vi "五参数水样测试.vi"(11 "启动参数":T1={"测量模式"=enum."水样测试", "数据标记表"="N", "测量时间"=3.0}) -> ()   [LabVIEW 2016, in "斯坦道多参数.lvlib"]
panel:
  out "枚举":T2(ring)
  out "状态":string
  out "数值":i32
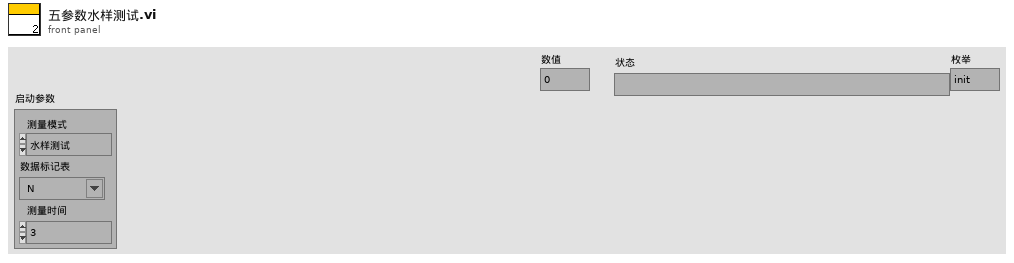
[diagram p1: front panel]
types:
  T1 = cluster{"测量模式":enum16{"待机", "水样测试", "标样核查", "零点核查", "跨度核查", "空白测试", "平行样测试", "加标回收", "空白校准", "标样校准", "初始化（清洗）"}, "数据标记表":string, "测量时间":dbl}
  T2 = enum16{"init", "开机", "启动测量", "读取测量值", "存储数据", "关闭测量", "关机", "结束"}
  T3 = cluster{"时间标识":timestamp, "设备":string, "日志信息":string, "流程参数":string}
  T4 = cluster{"系统时间":timestamp, "工作状态":u16, "测量模式":u16, "告警代码":enum16{"无告警", "缺试剂告警", "缺水样告警", "缺蒸馏水告警", "缺标液告警", "仪表漏液告警", "标定异常告警", "超量程告警", "加热异常", "低试剂预警", "超上限告警", "超下限告警", "仪表内部其他异常", "滴定异常告警", "电极异常告警", "量程切换告警", "参数设置告警", "PH电极电位异常", "电导率电极异常", "浊度光度异常", "溶解氧电极异常", "溶解氧光强异常", "温度异常告警", "PH异常告警", "溶解氧异常告警", "电导率异常告警", "浊度异常告警", "叶绿素异常告警", "藻密度异常告警", "蓝绿藻异常告警", "ORP异常告警", "氨氮异常告警", "清洁刷异常告警", "SD卡异常告警", "蓝牙异常告警", "Wifi异常告警", "流程异常告警"}, "故障代码":enum16{"无故障", "电机故障", "温度故障", "通讯故障", "滴定故障"}, "日志代码":u16, "软件版本":string}
  T5 = enum16{"待机", "水样测试", "标样核查", "零点核查", "跨度核查", "空白测试", "平行样测试", "加标回收", "空白校准", "标样校准", "初始化（清洗）"}
  T6 = cluster{"水温":dbl, "pH":dbl, "DO":dbl, "Cond":dbl, "Turb":dbl, "叶绿素":dbl, "藻密度":dbl, "蓝绿藻":dbl, "ORP":dbl, "NH3N":dbl}
  T7 = cluster{"数据标记表":string, "测量模式":enum16{"待机", "水样测试", "标样核查", "零点核查", "跨度核查", "空白测试", "平行样测试", "加标回收", "空白校准", "标样校准", "初始化（清洗）"}, "database":string}
  T8 = cluster{"因子编码":string, "单位":string, "标样参考值":sgl, "水样数据时间":timestamp, "水样实测值":sgl, "水样数据标识":string, "K":sgl, "B":sgl, "T":sgl, "H":sgl, "水深":sgl, "探头温度":sgl}
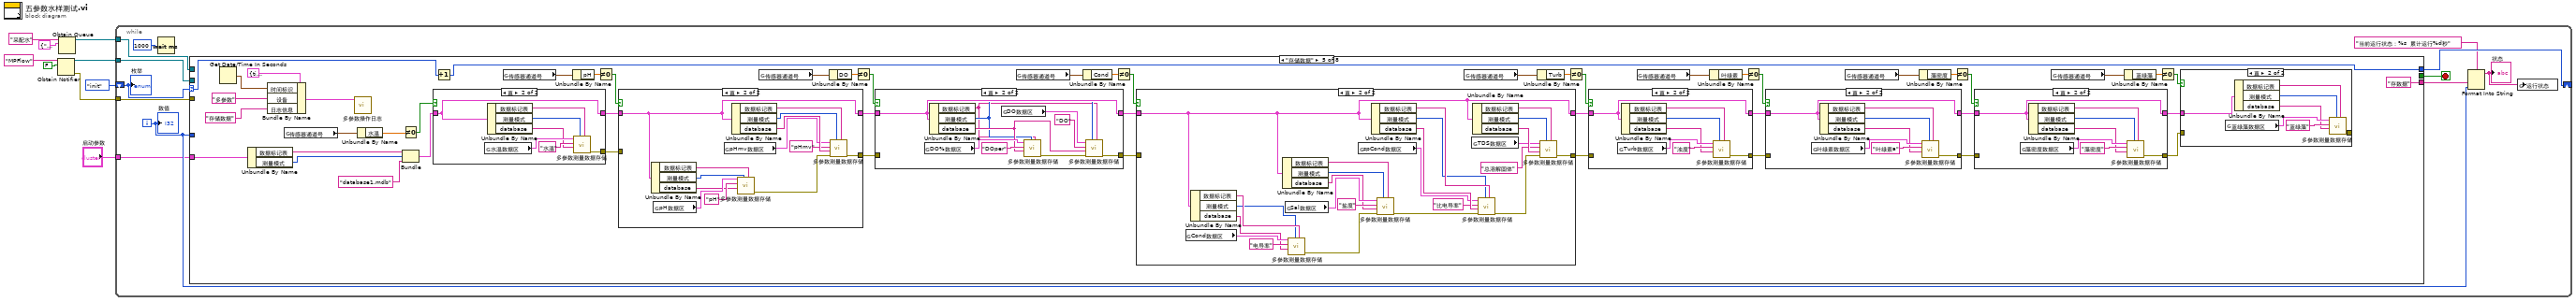
[diagram p0: block diagram]
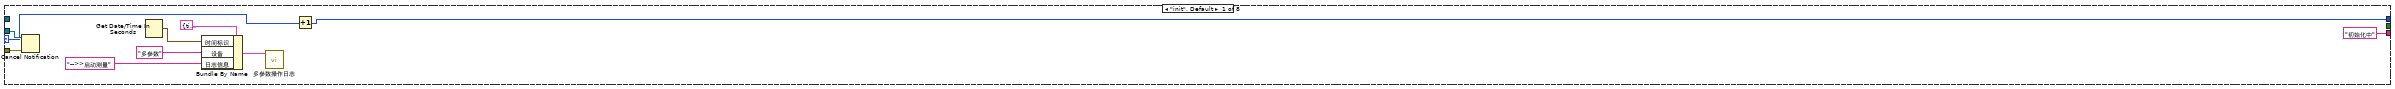
[diagram p2: hidden frame]
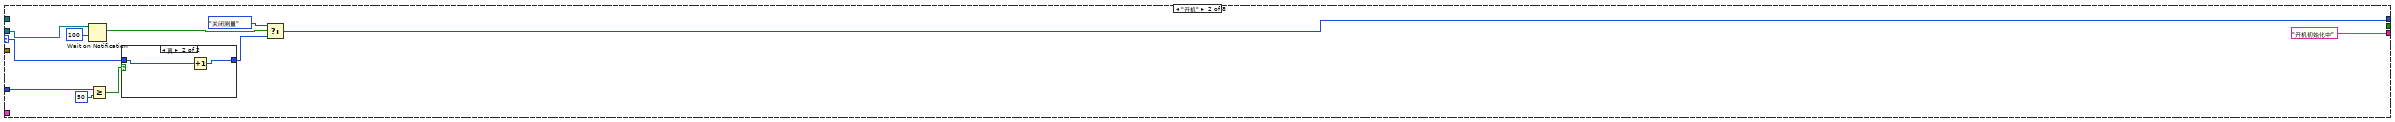
[diagram p3: hidden frame]
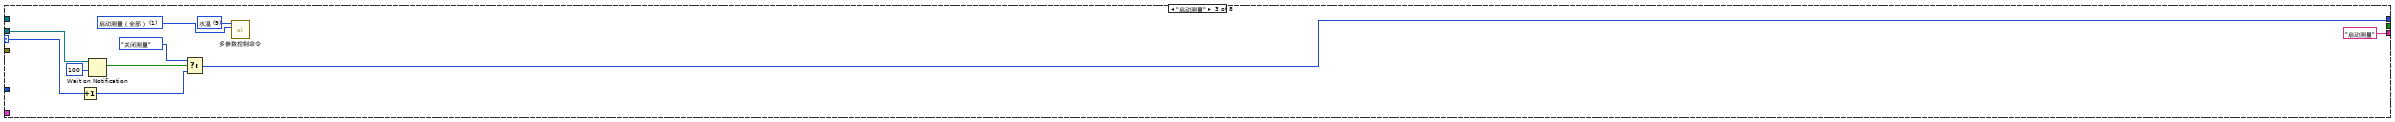
[diagram p5: hidden frame]
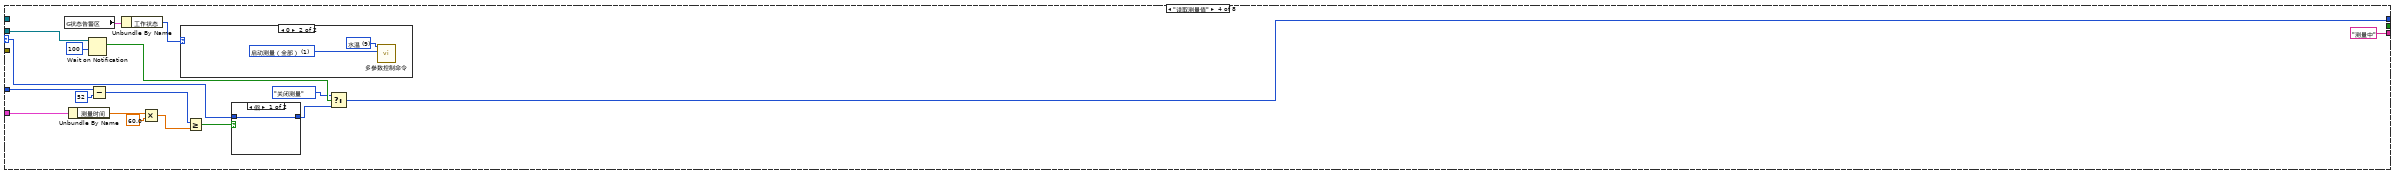
[diagram p6: hidden frame]
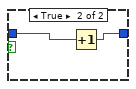
[diagram p8: hidden frame]
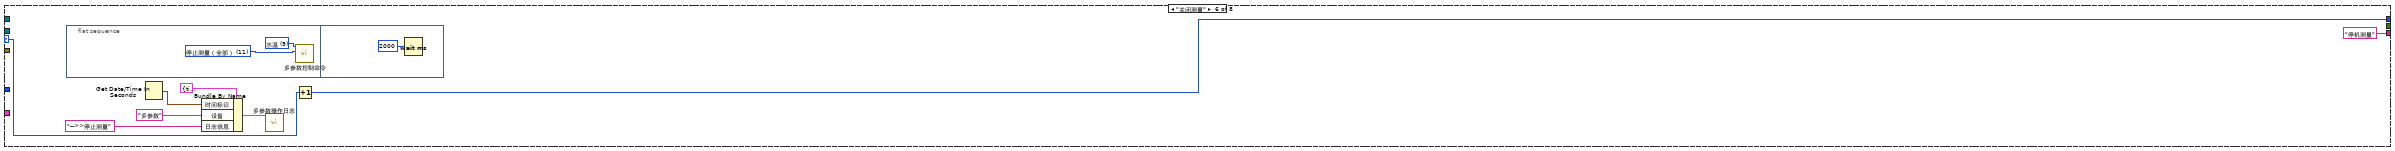
[diagram p17: hidden frame]
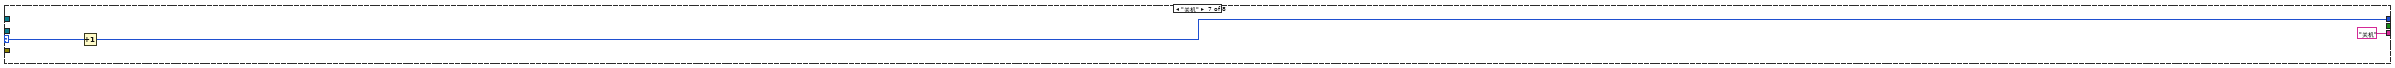
[diagram p18: hidden frame]
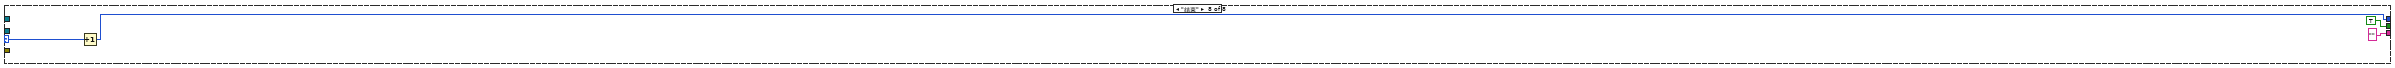
[diagram p19: hidden frame]
diagram:
  n1 = Obtain Notifier(name (unnamed)="MPFlow" ("名称（未命名）"), notification data type=FALSE) -> (notifier out=w6:refnum<notifier>, error out=w5:errorcluster)  [unwired: 2 in, 1 out]
  n2 = Obtain Queue(name (unnamed)="采配水" ("名称（未命名）"), element data type=cluster{"命令":string, "数据":variant} {"命令"="", "数据"=variant}) -> (queue out=w1:refnum<queue>)  [unwired: 3 in, 2 out]
  n3 = while {
    shift-right: [w17] -> _
    shift-left: T2."init" ("枚举") -> [w21]
    tunnel: w6 -> [w19]
    tunnel: w5 -> [w18]
    tunnel: "启动参数" -> [w11]
    tunnel: w1 -> [w10]
    i -> [w13]
    stop <- w20 stop-if-true
    n4 = Wait (ms)(milliseconds to wait=u32 1000 ("等待时间（毫秒）")) -> ()  [unwired: 1 out]
    n5 = case shown="\"存储数据\"" w21 {
      selector: w21 -> [w29 w42 w55 w73 w129 w227 w233 w236]
      tunnel: [_ _ _ _ _ _ _ TRUE] -> w20
      tunnel: w19 -> [w31 w37 w54 w70 _ _ _ _]
      tunnel: w18 -> [w30 _ _ _ _ _ _ _]
      tunnel: [w28 w35 w51 w68 w128 w226 w232 w235] -> w17
      tunnel: w13 -> [_ w41 _ w60 _ _ _ _]
      tunnel: ["初始化中" ("状态") "开机初始化中" ("状态") "启动测量" ("状态") "测量中" ("状态") "存数据" ("状态") "停机测量" ("状态") "关机" ("状态") "" ("状态")] -> w14
      tunnel: w11 -> [_ _ _ w64 w126 _ _ _]
      tunnel: w10 -> [_ _ _ _ _ _ _ _]
      frame "init", Default {
        n6 = Cancel Notification(0:w31, 3:w30) -> ()  [unwired: 3 out]
        n7 = Get Date/Time In Seconds() -> (seconds since 1Jan1904=w25:timestamp)
        n8 = Bundle By Name(cluster=T3 {"时间标识"=timestamp(0 s since 1904-01-01), "设备"="", "日志信息"="", "流程参数"=""} ("data in"), "时间标识"=w25, "设备"="多参数", "日志信息"="-->>启动测量") -> (w24:T3)
        n9 = call "多参数操作日志.vi"("data in"=w24) -> ()  [unwired: 10 in, 1 out]
        n10 = Increment(x=w29) -> (x+1=w28:T2)
      }
      frame "开机" {
        n11 = Wait on Notification(notifier=w37, timeout in ms (-1)=100 ("超时毫秒(-1)")) -> (notification=w38:bool)  [unwired: 2 in, 3 out]
        n12 = Greater Or Equal?(x=w41, y=50) -> (x >= y?=w39:bool)
        n13 = case shown="真" w39 {
          tunnel: w42 -> [w43 w45]
          tunnel: [w43 w44] -> w36
          frame False {
          }
          frame True {
            n14 = Increment(x=w45) -> (x+1=w44:T2)
          }
        }
        n15 = Select(t=T2."关闭测量" ("枚举"), s=w38, f=w36) -> (s? t:f=w35:T2)
      }
      frame "启动测量" {
        w46 = u16 1 items=["启动测量（全部）"=1, "初始化（清洗）"=10, "停止测量（全部）"=11, "校时"=13, "启动测量（单个传感器）"=19, "停止测量（单个传感器）"=20] ("控制命令")
        w47 = u16 9 items=["氨氮"=3, "水温"=9, "pH值"=10, "溶解氧"=11, "电导率"=12, "浊度"=13, "叶绿素a"=14, "藻密度"=15, "蓝绿藻"=16, "氧化还原电位"=17, "溶解氧%"=18, "盐度"=19] ("站号")
        n16 = Increment(x=w55) -> (x+1=w52:T2)
        n17 = Wait on Notification(notifier=w54, timeout in ms (-1)=100 ("超时毫秒(-1)")) -> (notification=w53:bool)  [unwired: 2 in, 3 out]
        n18 = Select(t=T2."关闭测量" ("枚举"), s=w53, f=w52) -> (s? t:f=w51:T2)
        n19 = call "多参数控制命令.vi"("控制命令"=w46, "站号"=w47) -> ()  [unwired: 9 in, 1 out]
      }
      frame "读取测量值" {
        n20 = global read "多参数全局变量.vi" "状态告警区"() -> (w57:T4)
        n21 = Unbundle By Name(w64) -> ("测量时间"=w63:dbl)
        n22 = Wait on Notification(notifier=w70, timeout in ms (-1)=100 ("超时毫秒(-1)")) -> (notification=w71:bool)  [unwired: 2 in, 3 out]
        n23 = Subtract(x=w60, y=52) -> (x-y=w59:i32)
        n24 = Unbundle By Name(w57) -> ("工作状态"=w56:u16)
        n25 = Multiply(x=w63, y=60.0) -> (x*y=w61:dbl)
        n26 = case shown="0" w56 {
          frame Default {
          }
          frame 0 {
            w74 = u16 1 items=["启动测量（全部）"=1, "初始化（清洗）"=10, "停止测量（全部）"=11, "校时"=13, "启动测量（单个传感器）"=19, "停止测量（单个传感器）"=20] ("控制命令")
            w75 = u16 9 items=["氨氮"=3, "水温"=9, "pH值"=10, "溶解氧"=11, "电导率"=12, "浊度"=13, "叶绿素a"=14, "藻密度"=15, "蓝绿藻"=16, "氧化还原电位"=17, "溶解氧%"=18, "盐度"=19] ("站号")
            n27 = call "多参数控制命令.vi"("控制命令"=w74, "站号"=w75) -> ()  [unwired: 9 in, 1 out]
          }
        }
        n28 = Greater Or Equal?(x=w59, y=w61) -> (x >= y?=w72:bool)
        n29 = case shown="假" w72 {
          tunnel: w73 -> [w76 w78]
          tunnel: [w76 w77] -> w69
          frame False {
          }
          frame True {
            n30 = Increment(x=w78) -> (x+1=w77:T2)
          }
        }
        n31 = Select(t=T2."关闭测量" ("枚举"), s=w71, f=w69) -> (s? t:f=w68:T2)
      }
      frame "存储数据" {
        n32 = Get Date/Time In Seconds() -> (seconds since 1Jan1904=w97:timestamp)
        n33 = Unbundle By Name(w126) -> ("数据标记表"=w105:string, "测量模式"=w104:T5)
        n34 = Bundle By Name(cluster=T3 {"时间标识"=timestamp(0 s since 1904-01-01), "设备"="", "日志信息"="", "流程参数"=""} ("data in"), "时间标识"=w97, "设备"="多参数", "日志信息"="存储数据") -> (w96:T3)
        n35 = global read "多参数全局变量.vi" "传感器通道号"() -> (w121:T6)
        n36 = call "多参数操作日志.vi"("data in"=w96) -> ()  [unwired: 10 in, 1 out]
        n37 = Unbundle By Name(w121) -> ("水温"=w120:dbl)
        n38 = Not Equal To 0?(x=w120) -> (x != 0?=w119:bool)
        n39 = Bundle("数据标记表"=w105, "测量模式"=w104, "database"="database1.mdb") -> (w103:T7)  [unwired: 1 in]
        n40 = case shown="真" w119 {
          tunnel: [_ w217] -> w125
          tunnel: w103 -> [w212 w216]
          tunnel: [w212 w216] -> w102
          frame False {
          }
          frame True {
            n41 = global read "多参数全局变量.vi" "水温数据区"() -> (w219:T8)
            n42 = Unbundle By Name(w216) -> ("数据标记表"=w215:string, "测量模式"=w214:T5, "database"=w213:string)
            n43 = call "多参数测量数据存储.vi"("数据标记表"=w215, "测量模式"=w214, "database"=w213, "table输入"="水温", "data in"=w219) -> ("error out"=w217:errorcluster)  [unwired: 6 in]
          }
        }
        n44 = Increment(x=w129) -> (x+1=w128:T2)
        n45 = global read "多参数全局变量.vi" "传感器通道号"() -> (w114:T6)
        n46 = Unbundle By Name(w114) -> ("pH"=w113:dbl)
        n47 = Not Equal To 0?(x=w113) -> (x != 0?=w118:bool)
        n48 = case shown="真" w118 {
          tunnel: w125 -> [_ _]
          tunnel: [_ w201] -> w124
          tunnel: w102 -> [w198 w206]
          tunnel: [w198 w206] -> w100
          frame False {
          }
          frame True {
            n49 = Unbundle By Name(w206) -> ("数据标记表"=w209:string, "测量模式"=w208:T5, "database"=w207:string)
            n50 = global read "多参数全局变量.vi" "pH数据区"() -> (w211:T8)
            n51 = global read "多参数全局变量.vi" "pHmv数据区"() -> (w200:T8)
            n52 = Unbundle By Name(w206) -> ("数据标记表"=w205:string, "测量模式"=w204:T5, "database"=w203:string)
            n53 = call "多参数测量数据存储.vi"("数据标记表"=w209, "测量模式"=w208, "database"=w207, "table输入"="pH", "data in"=w211) -> ("error out"=w202:errorcluster)  [unwired: 6 in]
            n54 = call "多参数测量数据存储.vi"("数据标记表"=w205, "测量模式"=w204, "error in (no error)"=w202, "database"=w203, "table输入"="pHmv", "data in"=w200) -> ("error out"=w201:errorcluster)  [unwired: 5 in]
          }
        }
        n55 = global read "多参数全局变量.vi" "传感器通道号"() -> (w112:T6)
        n56 = Unbundle By Name(w112) -> ("DO"=w111:dbl)
        n57 = Not Equal To 0?(x=w111) -> (x != 0?=w117:bool)
        n58 = case shown="真" w117 {
          tunnel: w124 -> [_ _]
          tunnel: [_ w194] -> w123
          tunnel: [w187 w191] -> w101
          tunnel: w100 -> [w187 w191]
          frame False {
          }
          frame True {
            n59 = global read "多参数全局变量.vi" "DO%数据区"() -> (w193:T8)
            n60 = Unbundle By Name(w191) -> ("数据标记表"=w188:string, "测量模式"=w189:T5, "database"=w190:string)
            n61 = global read "多参数全局变量.vi" "DO数据区"() -> (w195:T8)
            n62 = call "多参数测量数据存储.vi"("数据标记表"=w188, "测量模式"=w189, "database"=w190, "table输入"="DOper", "data in"=w193) -> ("error out"=w197:errorcluster)  [unwired: 6 in]
            n63 = call "多参数测量数据存储.vi"("数据标记表"=w188, "测量模式"=w189, "error in (no error)"=w197, "database"=w190, "table输入"="DO", "data in"=w195) -> ("error out"=w194:errorcluster)  [unwired: 5 in]
          }
        }
        n64 = global read "多参数全局变量.vi" "传感器通道号"() -> (w110:T6)
        n65 = Unbundle By Name(w110) -> ("Cond"=w109:dbl)
        n66 = Not Equal To 0?(x=w109) -> (x != 0?=w116:bool)
        n67 = case shown="真" w116 {
          tunnel: w123 -> [_ _]
          tunnel: [_ w166] -> w122
          tunnel: w101 -> [w161 w175]
          tunnel: [w161 w175] -> w99
          frame False {
          }
          frame True {
            n68 = global read "多参数全局变量.vi" "Cond数据区"() -> (w186:T8)
            n69 = Unbundle By Name(w175) -> ("数据标记表"=w180:string, "测量模式"=w179:T5, "database"=w181:string)
            n70 = Unbundle By Name(w175) -> ("数据标记表"=w178:string, "测量模式"=w177:T5, "database"=w176:string)
            n71 = global read "多参数全局变量.vi" "Sal数据区"() -> (w183:T8)
            n72 = call "多参数测量数据存储.vi"("数据标记表"=w180, "测量模式"=w179, "database"=w181, "table输入"="电导率", "data in"=w186) -> ("error out"=w184:errorcluster)  [unwired: 6 in]
            n73 = global read "多参数全局变量.vi" "spCond数据区"() -> (w165:T8)
            n74 = Unbundle By Name(w175) -> ("数据标记表"=w174:string, "测量模式"=w173:T5, "database"=w172:string)
            n75 = call "多参数测量数据存储.vi"("数据标记表"=w178, "测量模式"=w177, "error in (no error)"=w184, "database"=w176, "table输入"="盐度", "data in"=w183) -> ("error out"=w171:errorcluster)  [unwired: 5 in]
            n76 = global read "多参数全局变量.vi" "TDS数据区"() -> (w164:T8)
            n77 = Unbundle By Name(w175) -> ("数据标记表"=w167:string, "测量模式"=w168:T5, "database"=w169:string)
            n78 = call "多参数测量数据存储.vi"("数据标记表"=w174, "测量模式"=w173, "error in (no error)"=w171, "database"=w172, "table输入"="比电导率", "data in"=w165) -> ("error out"=w170:errorcluster)  [unwired: 5 in]
            n79 = call "多参数测量数据存储.vi"("数据标记表"=w167, "测量模式"=w168, "error in (no error)"=w170, "database"=w169, "table输入"="总溶解固体", "data in"=w164) -> ("error out"=w166:errorcluster)  [unwired: 5 in]
          }
        }
        n80 = global read "多参数全局变量.vi" "传感器通道号"() -> (w108:T6)
        n81 = Unbundle By Name(w108) -> ("Turb"=w107:dbl)
        n82 = Not Equal To 0?(x=w107) -> (x != 0?=w115:bool)
        n83 = case shown="真" w115 {
          tunnel: w122 -> [_ _]
          tunnel: w99 -> [w153 w154]
          tunnel: [_ w155] -> w90
          tunnel: [w153 w154] -> w89
          frame False {
          }
          frame True {
            n84 = global read "多参数全局变量.vi" "Turb数据区"() -> (w160:T8)
            n85 = Unbundle By Name(w154) -> ("数据标记表"=w156:string, "测量模式"=w157:T5, "database"=w158:string)
            n86 = call "多参数测量数据存储.vi"("数据标记表"=w156, "测量模式"=w157, "database"=w158, "table输入"="浊度", "data in"=w160) -> ("error out"=w155:errorcluster)  [unwired: 6 in]
          }
        }
        n87 = global read "多参数全局变量.vi" "传感器通道号"() -> (w92:T6)
        n88 = Unbundle By Name(w92) -> ("叶绿素"=w93:dbl)
        n89 = Not Equal To 0?(x=w93) -> (x != 0?=w91:bool)
        n90 = case shown="真" w91 {
          tunnel: w90 -> [_ _]
          tunnel: w89 -> [w145 w146]
          tunnel: [_ w147] -> w85
          tunnel: [w145 w146] -> w84
          frame False {
          }
          frame True {
            n91 = global read "多参数全局变量.vi" "叶绿素数据区"() -> (w152:T8)
            n92 = Unbundle By Name(w146) -> ("数据标记表"=w148:string, "测量模式"=w149:T5, "database"=w150:string)
            n93 = call "多参数测量数据存储.vi"("数据标记表"=w148, "测量模式"=w149, "database"=w150, "table输入"="叶绿素a", "data in"=w152) -> ("error out"=w147:errorcluster)  [unwired: 6 in]
          }
        }
        n94 = global read "多参数全局变量.vi" "传感器通道号"() -> (w87:T6)
        n95 = Unbundle By Name(w87) -> ("藻密度"=w86:dbl)
        n96 = Not Equal To 0?(x=w86) -> (x != 0?=w88:bool)
        n97 = case shown="真" w88 {
          tunnel: w85 -> [_ _]
          tunnel: w84 -> [w137 w139]
          tunnel: [w137 w139] -> w80
          tunnel: [_ w138] -> w79
          frame False {
          }
          frame True {
            n98 = global read "多参数全局变量.vi" "藻密度数据区"() -> (w144:T8)
            n99 = Unbundle By Name(w139) -> ("数据标记表"=w140:string, "测量模式"=w141:T5, "database"=w142:string)
            n100 = call "多参数测量数据存储.vi"("数据标记表"=w140, "测量模式"=w141, "database"=w142, "table输入"="藻密度", "data in"=w144) -> ("error out"=w138:errorcluster)  [unwired: 6 in]
          }
        }
        n101 = global read "多参数全局变量.vi" "传感器通道号"() -> (w82:T6)
        n102 = Unbundle By Name(w82) -> ("蓝绿藻"=w83:dbl)
        n103 = Not Equal To 0?(x=w83) -> (x != 0?=w81:bool)
        n104 = case shown="真" w81 {
          tunnel: w79 -> [_ _]
          tunnel: w80 -> [_ w134]
          tunnel: [_ w130] -> _
          frame False {
          }
          frame True {
            n105 = global read "多参数全局变量.vi" "蓝绿藻数据区"() -> (w136:T8)
            n106 = Unbundle By Name(w134) -> ("数据标记表"=w131:string, "测量模式"=w132:T5, "database"=w133:string)
            n107 = call "多参数测量数据存储.vi"("数据标记表"=w131, "测量模式"=w132, "database"=w133, "table输入"="蓝绿藻", "data in"=w136) -> ("error out"=w130:errorcluster)  [unwired: 6 in]
          }
        }
      }
      frame "关闭测量" {
        n108 = flat-sequence {
          frame #0 {
            w228 = u16 11 items=["启动测量（全部）"=1, "初始化（清洗）"=10, "停止测量（全部）"=11, "校时"=13, "启动测量（单个传感器）"=19, "停止测量（单个传感器）"=20] ("控制命令")
            w229 = u16 9 items=["氨氮"=3, "水温"=9, "pH值"=10, "溶解氧"=11, "电导率"=12, "浊度"=13, "叶绿素a"=14, "藻密度"=15, "蓝绿藻"=16, "氧化还原电位"=17, "溶解氧%"=18, "盐度"=19] ("站号")
            n109 = call "多参数控制命令.vi"("控制命令"=w228, "站号"=w229) -> ()  [unwired: 9 in, 1 out]
          }
          frame #1 {
            n110 = Wait (ms)(milliseconds to wait=u32 2000 ("等待时间（毫秒）")) -> ()  [unwired: 1 out]
          }
        }
        n111 = Get Date/Time In Seconds() -> (seconds since 1Jan1904=w223:timestamp)
        n112 = Bundle By Name(cluster=T3 {"时间标识"=timestamp(0 s since 1904-01-01), "设备"="", "日志信息"="", "流程参数"=""} ("data in"), "时间标识"=w223, "设备"="多参数", "日志信息"="-->>停止测量") -> (w222:T3)
        n113 = call "多参数操作日志.vi"("data in"=w222) -> ()  [unwired: 10 in, 1 out]
        n114 = Increment(x=w227) -> (x+1=w226:T2)
      }
      frame "关机" {
        n115 = Increment(x=w233) -> (x+1=w232:T2)
      }
      frame "结束" {
        n116 = Increment(x=w236) -> (x+1=w235:T2)
      }
    }
    n117 = Format Into String(format string="当前运行状态：%s  累计运行%d秒" ("格式字符串"), w14, w13) -> (resulting string=w12:string)  [unwired: 2 in, 1 out]
    "状态" <- w12
    n118 = global write "多参数全局变量.vi" "运行状态"(w12) -> ()
    "数值" <- w13
    "枚举" <- w21
  }
